vi "Tool information.vi"(7 "Tool in":T1, 11 "error in (no error)":errorcluster) -> (6 "Tool (folder) name":string, 8 "Main node address":u8, 10 "Expected stat 2 message len":u8, 15 "error out":errorcluster)   [LabVIEW 2011]
uses:
  List of tools.ctl
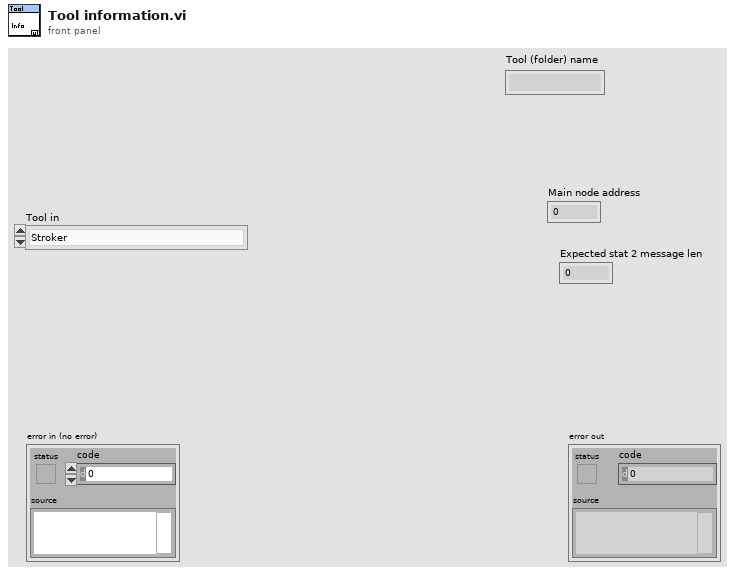
[diagram p1: front panel]
types:
  T1 = typedef "List of tools.ctl" = enum16{"Stroker", "Driller", "Tractor"}
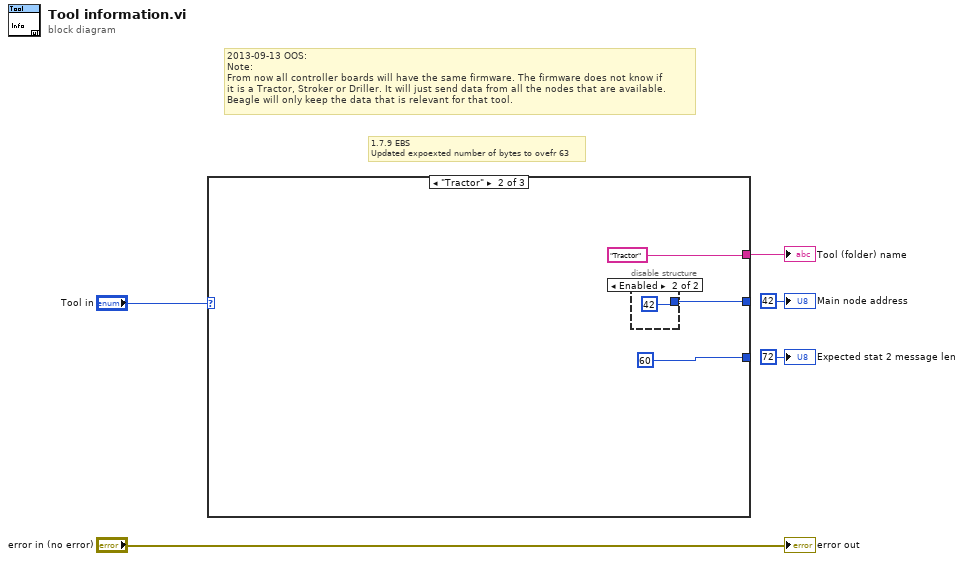
[diagram p0: block diagram]
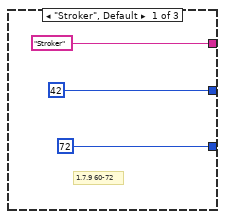
[diagram p2: hidden frame]
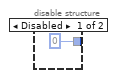
[diagram p3: hidden frame]
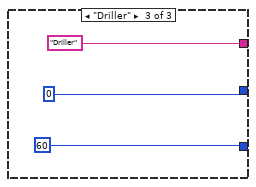
[diagram p4: hidden frame]
diagram:
  # "2013-09-13 OOS:\nNote: \nFrom now all controller boards will have the same firmware. The firmware does not know if\nit is a Tractor, Stroker or Driller. It will just send data from all the nodes that are available. \nBeagle will only keep the data that is relevant for that tool."
  # "1.7.9 EBS\nUpdated expoexted number of bytes to ovefr 63"
  n1 = case shown="\"Tractor\"" "Tool in" {
    tunnel: ["Stroker" ("Tool folder name") "Tractor" ("Tool folder name") "Driller" ("Tool folder name")] -> w3
    tunnel: [u8 42 ("Main node address") w10 u8 0 ("Main node address")] -> _
    tunnel: [u8 72 ("Expected message len") u8 60 ("Expected message len") u8 60 ("Expected message len")] -> _
    frame "Stroker", Default {
      # "1.7.9 60-72"
    }
    frame "Tractor" {
      n2 = disable-structure shown="Enabled" {
        disable-tunnel: [u8 0 ("Main node address") u8 42 ("Main node address")] -> w10
        frame Disabled {
        }
        frame Enabled {
        }
      }
    }
    frame "Driller" {
    }
  }
  "Tool (folder) name" <- w3
  "error out" <- "error in (no error)"
  "Main node address" <- u8 42 ("Main node address")
  "Expected stat 2 message len" <- u8 72 ("Expected message len")
